vi "set_value_from_eDoc_by_name.vi"(5 "little-endian?":bool, 8 "error in (no error)":errorcluster, 10 "arrayOfElements":T1[](array[typedef]), 11 "dataType in":variant) -> (0 "error out":errorcluster, 3 "Data dup":variant)   [LabVIEW 2015, in "BSON_convertors_Library.lvlib"]
doc: "Created by Artem Shevelev\nLabVIEW Portal profile: http://www.labviewportal.org/memberlist.php?mode=viewprofile&u=2340\ne-mail: artem.sh@gmail.com\nshevelev.pro"
uses:
  BSON_convertors_Library.lvlib
  typedefs/BSONelement.ctl
  typedefs/dataType.ctl
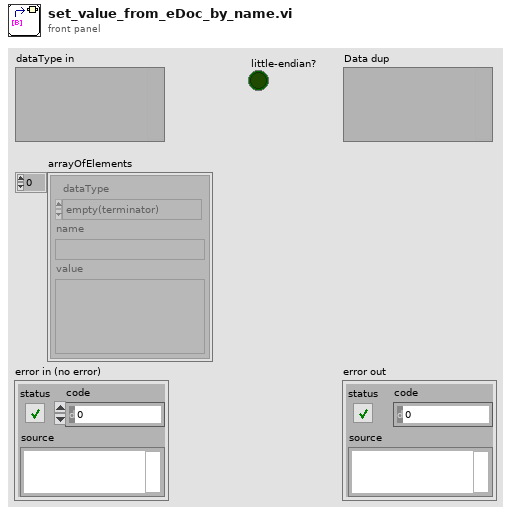
[diagram p1: front panel]
types:
  T1 = typedef "BSON_convertors_Library.lvlib/BSONelement.ctl" = cluster{"dataType":T2, "name":string, "value":variant}
  T2 = typedef "BSON_convertors_Library.lvlib/dataType.ctl" = enum8{"empty(terminator)", "double", "string", "document", "array", "binary", "Deprecated(Undefined)", "ObjectId", "boolean", "UTC datetime", "Null value", "cstring", "Deprecated(DBPointer)", "JavaScript", "Deprecated(Symbol)", "code_w_s", "int32", "uint64", "int64", "ext (decimal128)", "Min key", "Max key"}
  T3 = typedef "BSON_convertors_Library.lvlib/binaryData_cluster.ctl" = cluster{"subType":u8, "byteArray":u8[]}
  T4 = typedef "Type Descriptor Enumeration__ogtk.ctl" = enum8{"<Null>", "I8", "I16", "I32", "I64", "U8", "U16", "U32", "U64", "SGL", "DBL", "EXT", "CSG", "CDB", "CXT", "0x0F", "0x10", "0x11", "0x12", "0x13", "0x14", "Enum U8", "Enum U16", "Enum U32", "Enum U64", "SGL PQ", "DBL PQ", "EXT PQ", "CSG PQ", "CDB PQ", "CXT PQ", "0x1F", "0x20", "Boolean", "0x22", "0x23", "0x24", "0x25", "0x26", "0x27", "0x28", "0x29", "0x2A", "0x2B", "0x2C", "0x2D", "0x2E", "0x2F", "String", "0x31", "Path", "Pict", "0x34", "0x35", "0x36", "DAQ", "0x38", "0x39", "0x3A", "0x3B", "0x3C", "0x3D", "0x3E", "0x3F", "Array", "0x41", "0x42", "0x43", "0x44", "0x45", "0x46", "0x47", "0x48", "0x49", "0x4A", "0x4B", "0x4C", "0x4D", "0x4E", "0x4F", "Cluster", "0x51", "0x52", "Variant", "Waveform", "0x55", "0x56", "0x57", "0x58", "0x59", "0x5A", "0x5B", "0x5C", "0x5D", "0x5E", "0x5F", "0x60", "0x61", "0x62", "0x63", "0x64", "0x65", "0x66", "0x67", "0x68", "0x69", "0x6A", "0x6B", "0x6C", "0x6D", "0x6E", "0x6F", "Refnum"}
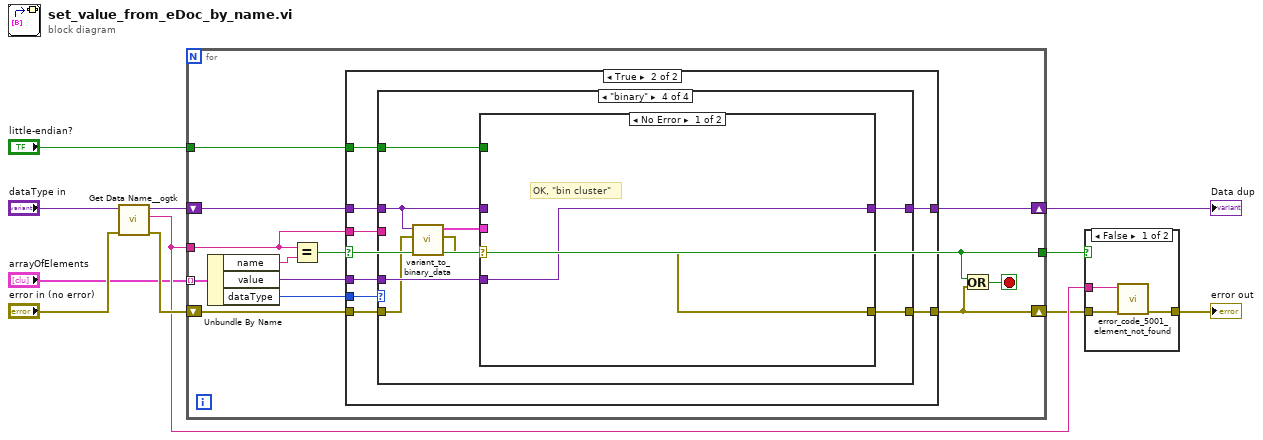
[diagram p0: block diagram]
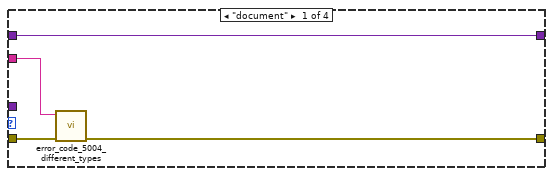
[diagram p4: hidden frame]
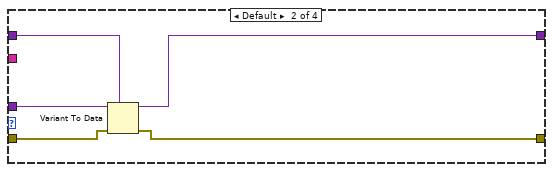
[diagram p5: hidden frame]
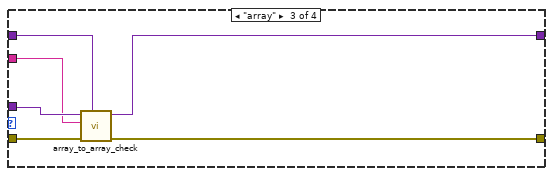
[diagram p6: hidden frame]
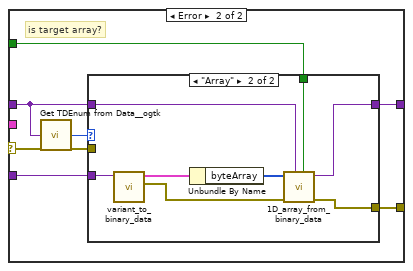
[diagram p7: hidden frame]
diagram:
  n1 = call <userlib>:"Get Data Name__ogtk.vi"("error in (no error)"="error in (no error)", "Data"="dataType in") -> ("error out"=w11:errorcluster, "Data Name"=w9:string, "Data dup"=w8:variant)  [unwired: 7 in]
  n2 = for {
    tunnel: "arrayOfElements" -> [w23] mode=indexing
    tunnel: w9 -> [w13]
    tunnel: [w16] -> w6
    shift-right: [w17] -> w5
    shift-left: w11 -> [w19]
    shift-right: [w15] -> w4
    shift-left: w8 -> [w20]
    tunnel: "little-endian?" -> [w12]
    stop <- w18 stop-if-true
    n3 = Unbundle By Name(w23) -> ("name"=w22:string, "value"=w21:variant, "dataType"=w14:T2)
    n4 = Equal?(x=w13, y=w22) -> (x = y?=w16:bool)
    n5 = case shown="True" w16 {
      tunnel: w21 -> [_ w33]
      tunnel: w20 -> [w25 w32]
      tunnel: [w25 w31] -> w15
      tunnel: w19 -> [w24 w30]
      tunnel: [w24 w29] -> w17
      tunnel: w14 -> [_ w28]
      tunnel: w13 -> [_ w27]
      tunnel: w12 -> [_ w26]
      frame False {
      }
      frame True {
        n6 = case shown="\"binary\"" w28 {
          tunnel: w33 -> [_ w42 w44 w55]
          tunnel: w32 -> [w34 w41 w46 w53]
          tunnel: [w34 w40 w45 w56] -> w31
          tunnel: w30 -> [w37 w39 w48 w50]
          tunnel: [w36 w38 w47 w54] -> w29
          tunnel: w27 -> [w35 _ w43 _]
          tunnel: w26 -> [_ _ _ w52]
          frame "document" {
            n7 = call "error_code_5004_different_types.vi"("error in (no error)"=w37, "name"=w35) -> ("error out"=w36:errorcluster)  [unwired: 9 in]
          }
          frame Default {
            n8 = Variant To Data(error in=w39, type=w41, Variant=w42) -> (data=w40:variant, error out=w38:errorcluster)
          }
          frame "array" {
            n9 = call "array_to_array_check.vi"("dataType"=w46, "error in (no error)"=w48, "name"=w43, "value in"=w44) -> ("error out"=w47:errorcluster, "value out"=w45:variant)  [unwired: 6 in]
          }
          frame "binary" {
            n10 = call "variant_to_binary_data.vi"("error in (no error)"=w50, "DataIn"=w53) -> ("error out"=w49:errorcluster, "binaryData"=w51:T3)  [unwired: 8 in]
            n11 = case shown="No Error" w49 {
              selector: w49 -> [w57 w61]
              tunnel: [w58 w60] -> w56
              tunnel: w55 -> [w58 w63]
              tunnel: [w57 w62] -> w54
              tunnel: w53 -> [_ w64]
              tunnel: w52 -> [_ w59]
              tunnel: w51 -> [_ _]
              frame No Error {
                # "OK, \"bin cluster\""
              }
              frame Error {
                # "is target array?"
                n12 = call <userlib>:"Get TDEnum from Data__ogtk.vi"("Data"=w64) -> ("Type Descriptor Enumeration"=w65:T4)  [unwired: 4 in]
                n13 = case shown="\"Array\"" w65 {
                  tunnel: w64 -> [w66 w75]
                  tunnel: w63 -> [_ w70]
                  tunnel: [w67 w72] -> w62
                  tunnel: w61 -> [w67 _]
                  tunnel: [w66 w73] -> w60
                  tunnel: w59 -> [_ w71]
                  frame Default {
                  }
                  frame "Array" {
                    n14 = call "variant_to_binary_data.vi"("DataIn"=w70) -> ("error out"=w68:errorcluster, "binaryData"=w69:T3)  [unwired: 9 in]
                    n15 = Unbundle By Name(w69) -> ("byteArray"=w74:u8[])
                    n16 = call "1D_array_from_binary_data.vi"("little-endian?"=w71, "inputArray(type)"=w75, "error in (no error)"=w68, "byteArray"=w74) -> ("error out"=w72:errorcluster, "dataArray"=w73:variant)  [unwired: 6 in]
                  }
                }
              }
            }
          }
        }
      }
    }
    n17 = Or(x=w16, y=w17) -> (x .or. y?=w18:bool)
  }
  "Data dup" <- w4
  n18 = case shown="False" w6 {
    tunnel: w5 -> [w78 w79]
    tunnel: w9 -> [w77 _]
    tunnel: [w76 w79] -> w7
    frame False {
      n19 = call "error_code_5001_element_not_found.vi"("error in (no error)"=w78, "name"=w77) -> ("error out"=w76:errorcluster)  [unwired: 9 in]
    }
    frame True {
    }
  }
  "error out" <- w7
